vi "Different Types.vi"() -> ()   [LabVIEW 2017, in "Assertions.Tests.lvlib" / "Assert Same Type.lvlib"]
uses:
  Assert Same Type.lvlib
  src/Transparent Assertions/Constraints/Is Same Type/Create.vi
  src/Transparent Assertions/Constraints/Is Same Type/Is Same Type.lvclass
  src/Transparent Assertions/Assertions/Assertions.lvlib
panel:
  out "error out":errorcluster
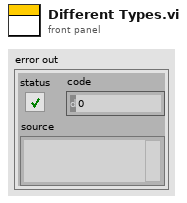
[diagram p1: front panel]
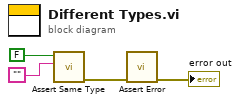
[diagram p0: block diagram]
diagram:
  n1 = call "Assert Same Type.vi"("Second"="", "First"=FALSE) -> ("error out"=w2:errorcluster)  [unwired: 9 in]
  n2 = call "Assert Error.vi"("error in (no error)"=w2) -> ("error out"=→"error out":errorcluster)  [unwired: 10 in]
